vi "meanAndVar.vi"(0 "new mean value":dbl, 2 "MEAN array in":dbl[](array[numeric]), 3 "VAR array in":dbl[](array[numeric])) -> (5 "arrays stack":dbl[][](array[numeric]), 6 "MEAN array out":dbl[](array[numeric]), 7 "VAR array out":dbl[](array[numeric]))   [LabVIEW 2023]
uses:
  <vilib>/Analysis/NI_AALBase.lvlib
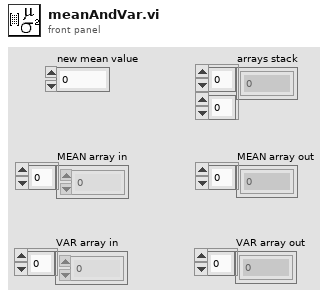
[diagram p1: front panel]
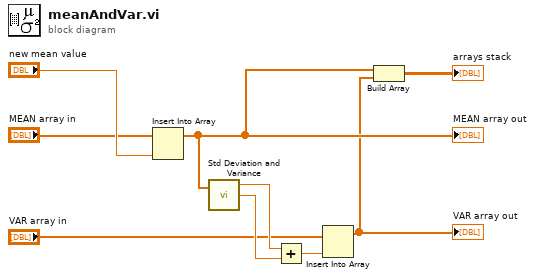
[diagram p0: block diagram]
diagram:
  n1 = Insert Into Array(array="MEAN array in", new element="new mean value") -> (w6:dbl[])  [unwired: 1 in]
  "MEAN array out" <- w6
  n2 = call <vilib>:"Std Deviation and Variance.vi"("X"=w6) -> ("mean"=w7:dbl, "standard deviation"=w8:dbl)  [unwired: 1 in, 1 out]
  n3 = Add(x=w7, y=w8) -> (x+y=w9:dbl)
  n4 = Insert Into Array(array="VAR array in", new element=w9) -> (w5:dbl[])  [unwired: 1 in]
  "VAR array out" <- w5
  n5 = Build Array(w6, w5) -> (→"arrays stack":dbl[][])
